vi "Word_Save_Document.vi"(0 "Word._Document":refnum<k7>, 5 "password":string, 7 "path":string, 11 "error in (no error)":errorcluster) -> (15 "error out":errorcluster)   [LabVIEW 2020, in "NI_ReportGenerationToolkit.lvlib"]
uses:
  <vilib>/addons/_office/NI_ReportGenerationToolkit.lvlib
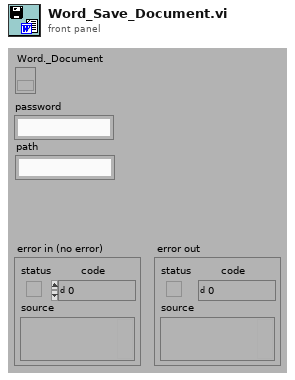
[diagram p1: front panel]
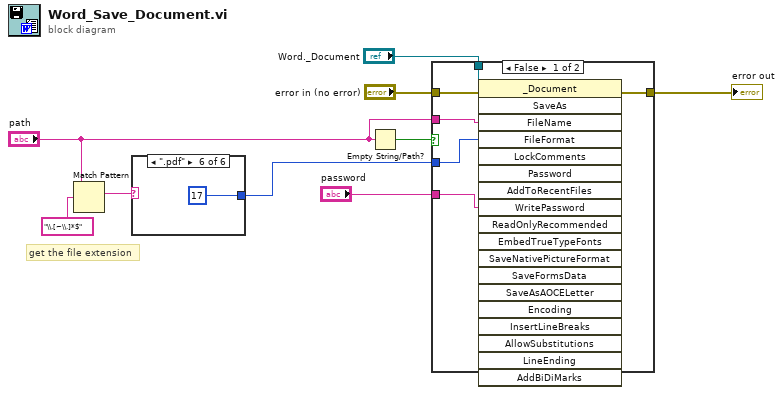
[diagram p0: block diagram]
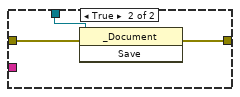
[diagram p2: hidden frame]
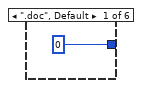
[diagram p3: hidden frame]
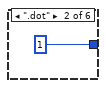
[diagram p4: hidden frame]
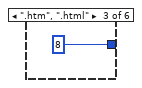
[diagram p5: hidden frame]
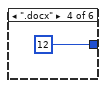
[diagram p6: hidden frame]
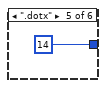
[diagram p7: hidden frame]
diagram:
  # "get the file extension"
  n1 = Match Pattern(string="path", regular expression="\\.[~\\.]*$") -> (match substring=w2:string)  [unwired: 4 out]
  n2 = case shown="\".pdf\"" w2 {
    tunnel: [0 1 8 12 14 17] -> w1
    frame ".doc", Default {
    }
    frame ".dot" {
    }
    frame ".htm", ".html" {
    }
    frame ".docx" {
    }
    frame ".dotx" {
    }
    frame ".pdf" {
    }
  }
  n3 = Empty String/Path?(string/path="path") -> (empty?=w6:bool)
  n4 = case shown="False" w6 {
    tunnel: "Word._Document" -> [w21 w24]
    tunnel: "path" -> [w17 _]
    tunnel: "error in (no error)" -> [w20 w23]
    tunnel: [w19 w22] -> w9
    tunnel: "password" -> [w18 _]
    tunnel: w1 -> [w16 _]
    frame False {
      n5 = invoke class="_Document" method="SaveAs"(reference=w21, error in=w20, "FileName"=w17, "FileFormat"=w16, "WritePassword"=w18) -> (error out=w19:errorcluster)  [unwired: 14 in, 18 out]
    }
    frame True {
      n6 = invoke class="_Document" method="Save"(reference=w24, error in=w23) -> (error out=w22:errorcluster)  [unwired: 1 in, 2 out]
    }
  }
  "error out" <- w9
